vi "Write.vi"(8 "error in (no error)":errorcluster, 10 "Log Data":T1={"Time"=timestamp(0 s since 1904-01-01), "Level"=enum."INFO", "Logger"="", "Message"="", "Arguments"=[]} {"Time" format="%<%x %.3X>T"}, 11 "Text File in":refnum<class "Text File.lvclass">) -> (0 "error out":errorcluster, 3 "Text File out":refnum<class "Text File.lvclass">)   [LabVIEW 2019, in "TSC Event Logger.lvlib" / "Text File.lvclass"]
uses:
  Text File.lvclass
  C:/Development/Reuse-libraries/Event Logger/Log Sinks/Log Sinks.lvclass
  Log Data.ctl
  Log/Event Level.ctl
  Text File.lvclass/Text File.ctl
  Log Sinks.lvclass
  TSC Event Logger.lvlib
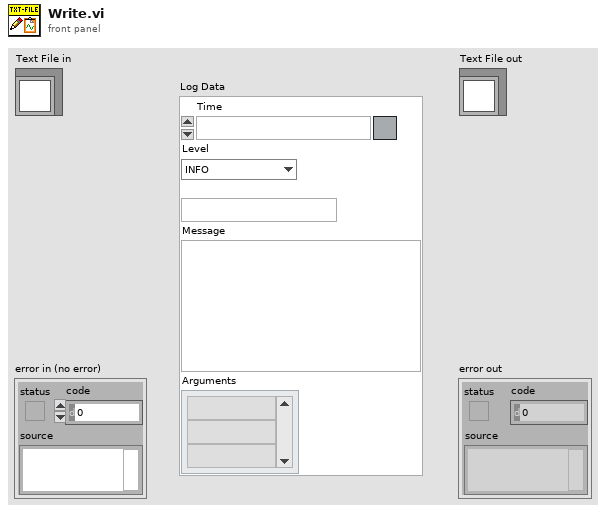
[diagram p1: front panel]
types:
  T1 = typedef "TSC Event Logger.lvlib/Log Data.ctl" = cluster{"Time":timestamp, "Level":T2, "Logger":string, "Message":string, "Arguments":string[]}
  T2 = typedef "TSC Event Logger.lvlib/Event Level.ctl" = enum16{"OFF", "TRACE", "DEBUG", "INFO", "WARN", "ERROR", "FATAL"}
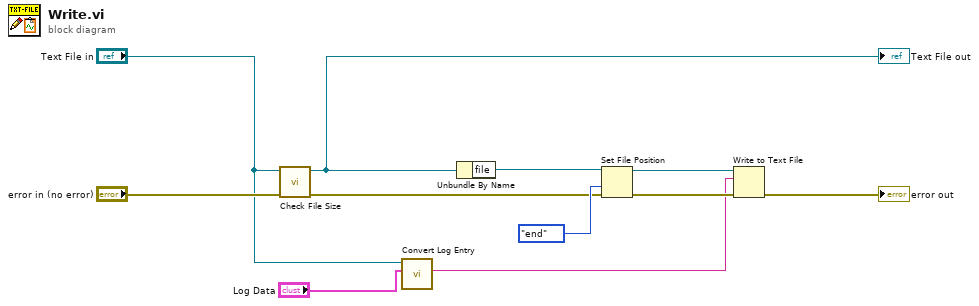
[diagram p0: block diagram]
diagram:
  n1 = call "Check File Size.vi"("error in (no error)"="error in (no error)", "Text File in"="Text File in") -> ("error out"=w6:errorcluster, "Text File out"=w1:refnum<class "Text File.lvclass">)  [unwired: 8 in]
  "Text File out" <- w1
  n2 = call "Convert Log Entry.vi"("Log Data"="Log Data", "Log Sink in"="Text File in") -> ("Log Entry"=w2:string)  [unwired: 9 in]
  n3 = Unbundle By Name(w1) -> ("file"=w5:refnum<file>)
  n4 = Set File Position(refnum=w5, from (0:start)=enum16{"start", "end", "current"}."end", error in=w6) -> (refnum out=w8:refnum<file>, error out=w11:errorcluster)  [unwired: 1 in]
  n5 = Write to Text File(file (use dialog)=w8, text=w2, error in=w11) -> (error out=→"error out":errorcluster)  [unwired: 1 in, 2 out]
